vi "End Configuration.vi"(8 "error in (no error)":errorcluster, 10 "GPIB Espectrometro":refnum<visa-resource-name>="GPIB0::9::INSTR", 11 "GPIB Controlador Laser Diodo":refnum<visa-resource-name>="GPIB0::1::INSTR") -> (0 "error out":errorcluster)   [LabVIEW 2021]
uses:
  a156afd7-33ea-40fc-bda6-a360d078db87.vi
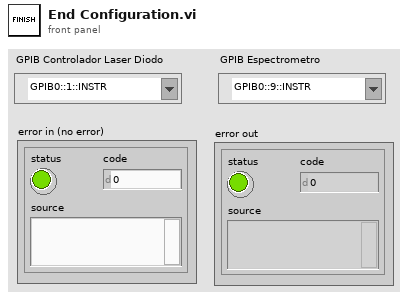
[diagram p1: front panel]
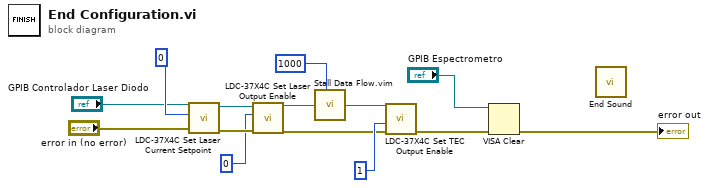
[diagram p0: block diagram]
diagram:
  n1 = call "LDC-37X4C Set Laser Current Setpoint.vi"("error in (no error)"="error in (no error)", "Current"=0, "VISA resource name"="GPIB Controlador Laser Diodo") -> ("error out"=w9:errorcluster, "VISA resource name out"=w10:refnum<visa-resource-name>)  [unwired: 7 in]
  n2 = call "LDC-37X4C Set Laser Output Enable.vi"("error in (no error)"=w9, "input 2"=0 ("input 1"), "VISA resource name"=w10) -> ("error out"=w8:errorcluster, "VISA resource name out"=w6:refnum<visa-resource-name>)  [unwired: 7 in]
  n3 = call "Stall Data Flow.vim"("value in"=w6, "milliseconds to wait"=u32 1000) -> ("value out"=w5:refnum<visa-resource-name>)  [unwired: 1 out]
  n4 = call "LDC-37X4C Set TEC Output Enable.vi"("error in (no error)"=w8, "input 1"=1, "VISA resource name"=w5) -> ("error out"=w2:errorcluster)  [unwired: 7 in, 1 out]
  n5 = VISA Clear(VISA resource name="GPIB Espectrometro", error in (no error)=w2) -> (error out=→"error out":errorcluster)  [unwired: 1 out]
  n6 = call "End Sound.vi"() -> ()  [unwired: 12 in]
